vi "clear Session Data.vi"(0 "Serial In":refnum<class "Serial Session.lvclass">, 11 "error in":errorcluster) -> (4 "Serial Out":refnum<class "Serial Session.lvclass">, 15 "error out":errorcluster)   [LabVIEW 2019, in "Serial Session.lvclass"]
doc: "OVERRIDE VI\nPlaceholder for decendant classes to clear session information and close references."
uses:
  Serial Session.lvclass
  Serial Session.lvclass/Serial Session.ctl
  Text Communication/Text Device Session.lvclass
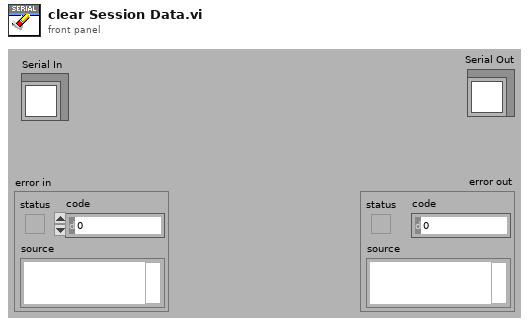
[diagram p1: front panel]
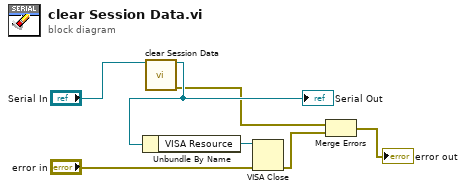
[diagram p0: block diagram]
diagram:
  n1 = call-parent "clear Session Data.vi"("OBJ - Measurement Session in"="Serial In") -> ("OBJ - Measurement Session out"=w4:refnum<class "Serial Session.lvclass">, "error out"=w1:errorcluster)  [unwired: 13 in]
  "Serial Out" <- w4
  n2 = Unbundle By Name(w4) -> ("VISA Resource"=w7:refnum<visa-resource-name>)
  n3 = VISA Close(VISA resource name=w7, error in (no error)="error in") -> (error out=w2:errorcluster)
  n4 = Merge Errors(w1, w2) -> (→"error out":errorcluster)
